vi "ReverseStringLines.vi"(5 "Lines in":string) -> (2 "Reversed Lines out":string)   [LabVIEW 2017]
doc: "Developed by Kevin Thompson\nkevin@thompsonengineering.net\n\nCopyright 2018-2020\nThompson Engineering, LLC"
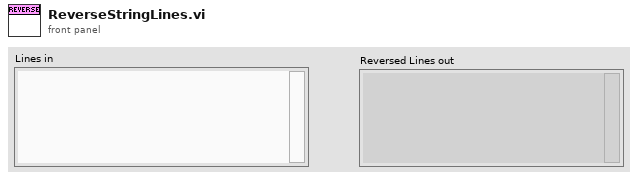
[diagram p1: front panel]
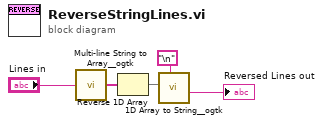
[diagram p0: block diagram]
diagram:
  n1 = call <userlib>:"Multi-line String to Array__ogtk.vi"("string"="Lines in") -> ("lines"=w2:string[])
  n2 = Reverse 1D Array(array=w2) -> (reversed array=w3:string[])
  n3 = call <userlib>:"1D Array to String__ogtk.vi"("delimiter (Tab)"="\n", "Array of Strings"=w3) -> ("delimited string"=→"Reversed Lines out":string)  [unwired: 9 in]
